vi "sequenceJsonIndex.vi"(8 "error in":errorcluster, 10 "StreamCluster":T1={"DAQ"={"ManagmentRate_Hz"=1, "StreamRate_Hz"=50, "StreamRate_ms"=20, "ManagmentRate_ms"=1000, "refDesArray"=[]}, "Modules"=[]}, 11 "JSON in":string) -> (0 "error out":errorcluster, 1 "refDes":string, 2 "cmd subset index":i32, 3 "cmd set index":i32)   [LabVIEW 2024]
uses:
  Control/StreamCluster_TypeDef.ctl
  c49e8bee-f697-436e-a8eb-f13d28c7991d.vi
  <vilib>/JDP Science/JSONtext/Find Item.vi
  <vilib>/JDP Science/JSONtext/Next JSON Value.vi
  <vilib>/JDP Science/JSONtext/String Subset.vi
  <vilib>/JDP Science/JSONtext/Parsing/Advance past next JSON Value (inlined COPY).vi
  <vilib>/JDP Science/JSONtext/Parsing/Advance past whitespace.vi
  <vilib>/JDP Science/JSONtext/Parsing/Advance past String.vi
  <vilib>/JDP Science/JSONtext/Parsing/Advance past Number.vi
  <vilib>/JDP Science/JSONtext/Parsing/Advance past Line Ending.vi
  <vilib>/JDP Science/JSONtext/Parsing/Parse Full Path or Item Name.vi
  <vilib>/JDP Science/JSONtext/Parsing/Advance past Array.vi
  <vilib>/JDP Science/JSONtext/Parsing/Advance past Object.vi
  <vilib>/JDP Science/JSONtext/support/Error Cluster From Code.vi
  <vilib>/JDP Science/JSONtext/Offset/Find Item Locations by Path.vi
  <vilib>/JDP Science/JSONtext/JSON text to Variant.vi
  <vilib>/JDP Science/JSONtext/LVClass Serializer/JSONtext LVClass Serializer.lvclass
  <vilib>/ErrorRing/Error Ring.xnode
  <vilib>/Utility/error.llb/Error Cluster From Error Code.vi
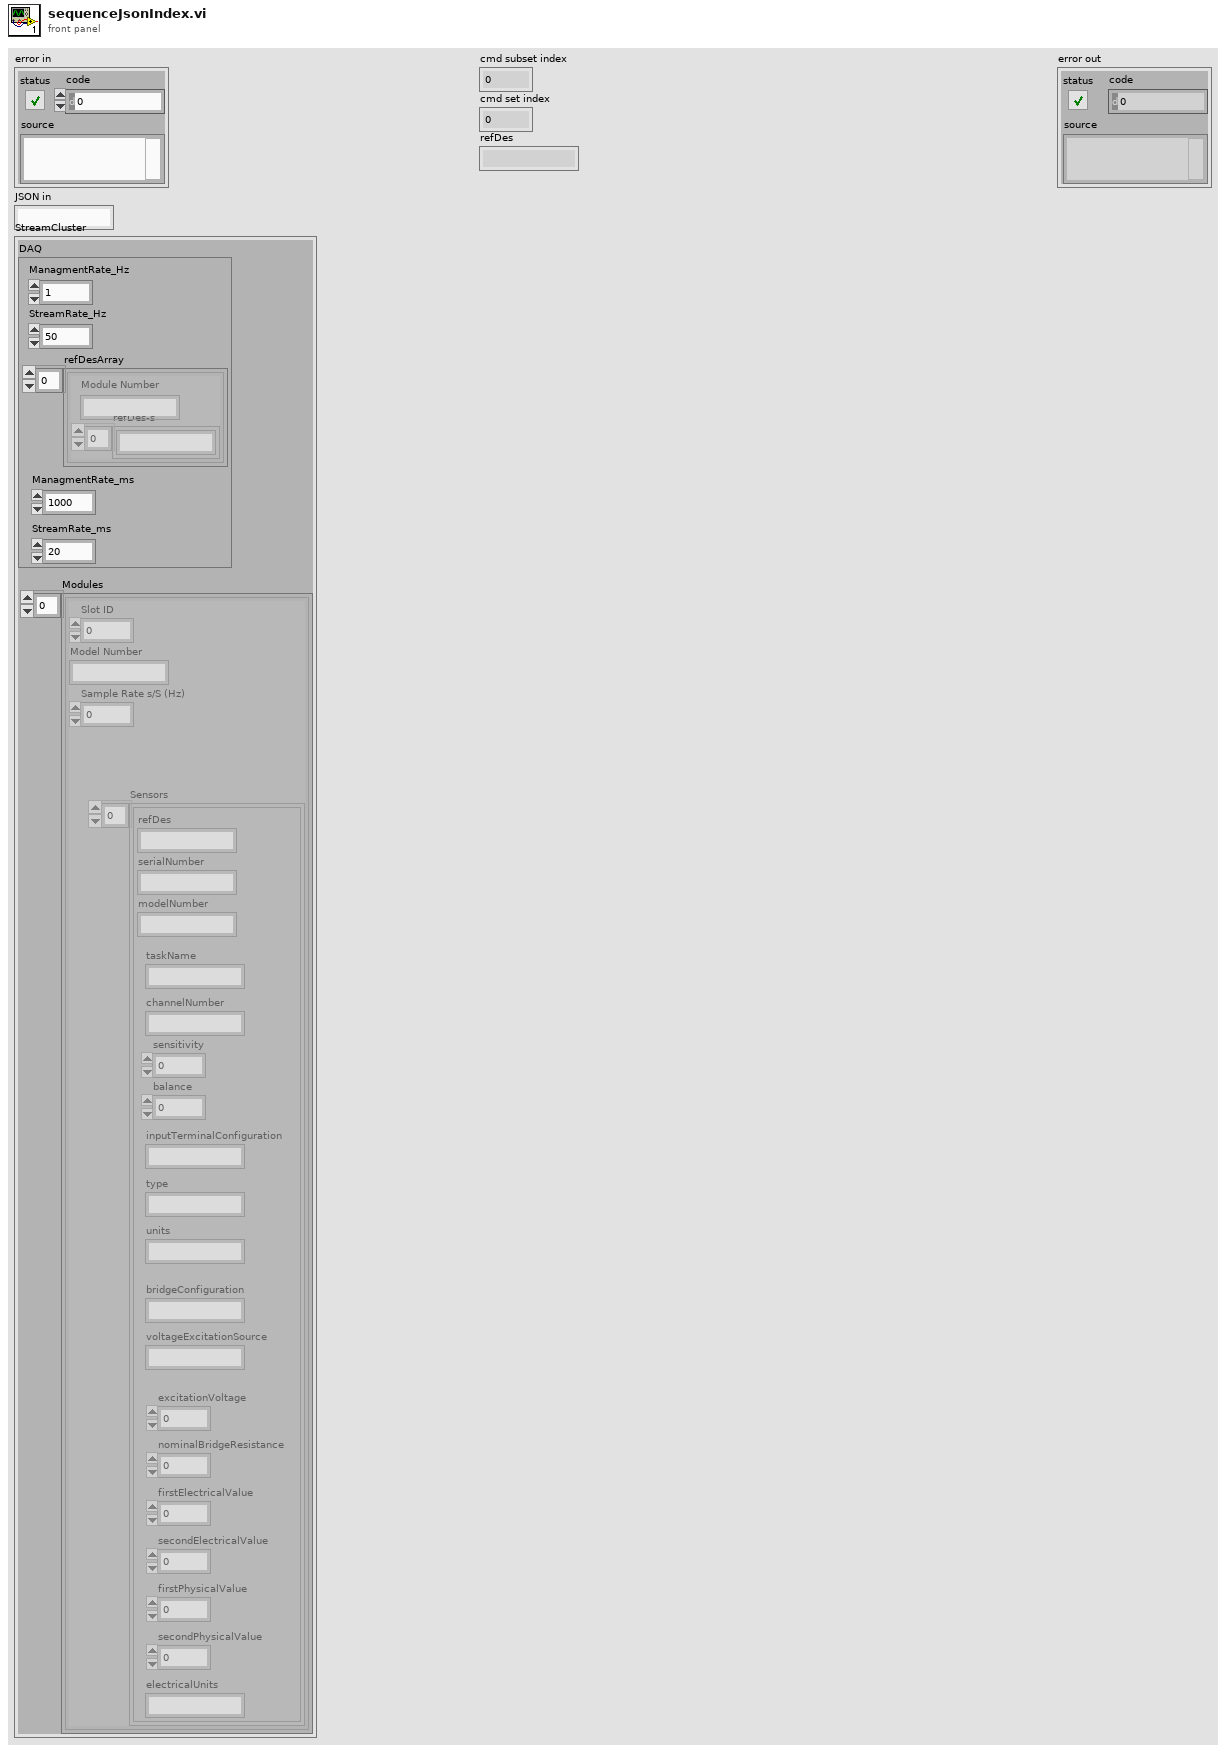
[diagram p1: front panel]
types:
  T1 = typedef "StreamCluster_TypeDef.ctl" = cluster{"DAQ":cluster{"ManagmentRate_Hz":i32, "StreamRate_Hz":i32, "StreamRate_ms":i32, "ManagmentRate_ms":i32, "refDesArray":cluster{"refDes-s":string[], "Module Number":string}[]}, "Modules":cluster{"Slot ID":i32, "Model Number":string, "Sample Rate s/S (Hz)":dbl, "Sensors":cluster{"refDes":string, "serialNumber":string, "modelNumber":string, "units":string, "balance":dbl, "sensitivity":dbl, "type":string, "inputTerminalConfiguration":string, "channelNumber":string, "taskName":string, "bridgeConfiguration":string, "excitationVoltage":dbl, "voltageExcitationSource":string, "nominalBridgeResistance":dbl, "firstElectricalValue":dbl, "secondElectricalValue":dbl, "firstPhysicalValue":dbl, "secondPhysicalValue":dbl, "electricalUnits":string}[]}[]}
  T2 = cluster{"refDes-s":string[], "Module Number":string}[]
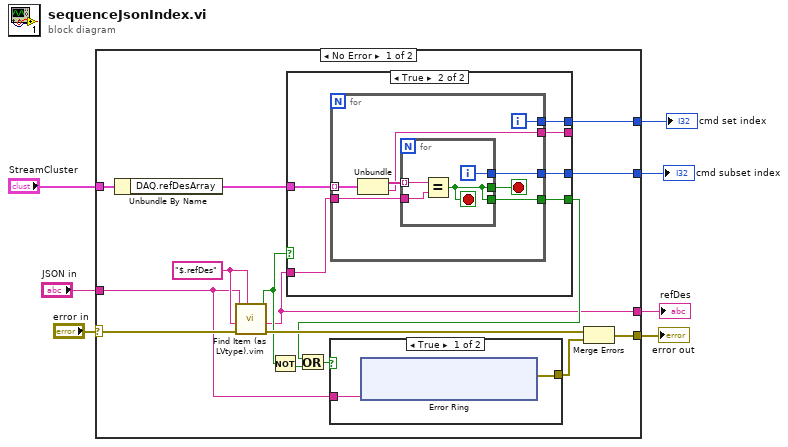
[diagram p0: block diagram]
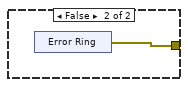
[diagram p2: hidden frame]
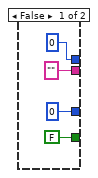
[diagram p3: hidden frame]
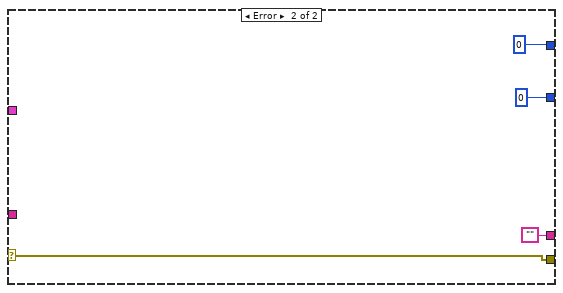
[diagram p4: hidden frame]
diagram:
  n1 = case shown="No Error" "error in" {
    selector: "error in" -> [w21 w59]
    tunnel: [w18 w59] -> w6
    tunnel: "JSON in" -> [w13 _]
    tunnel: "StreamCluster" -> [w20 _]
    tunnel: [w16 0] -> w3
    tunnel: [w15 0] -> w2
    tunnel: [w8 ""] -> w1
    frame No Error {
      w22 = "$.refDes" ("$Path or Item Name")
      n2 = Unbundle By Name(w20) -> ("DAQ.refDesArray"=w17:T2)
      n3 = call "Find Item (as LVtype).vim"("$Path or Item Name"=w22, "error in (no error)"=w21, "Data Type and Default Value"=w22, "JSON"=w13) -> ("error out"=w19:errorcluster, "Data"=w8:string, "Found"=w12:bool)  [unwired: 4 in, 1 out]
      n4 = Not(x=w12) -> (.not. x?=w10:bool)
      n5 = case shown="True" w12 {
        tunnel: w8 -> [_ w43]
        tunnel: w17 -> [_ w42]
        tunnel: [0 w41] -> w16
        tunnel: [0 w40] -> w15
        tunnel: [FALSE w39] -> w9
        tunnel: ["" ("Module Number") w38] -> _
        frame False {
        }
        frame True {
          n6 = for {
            tunnel: w43 -> [w49]
            tunnel: w42 -> [w51] mode=indexing
            tunnel: [w47] -> w39
            tunnel: [w46] -> w41
            tunnel: [w45] -> w40
            tunnel: [w44] -> w38
            i -> [w45]
            stop <- w48 stop-if-true
            n7 = Unbundle(w51) -> ("refDes-s"=w50:string[], "Module Number"=w44:string)
            n8 = for {
              tunnel: w50 -> [w55] mode=indexing
              tunnel: w49 -> [w54]
              tunnel: [w53] -> w48
              tunnel: [w53] -> w47
              tunnel: [w52] -> w46
              i -> [w52]
              stop <- w53 stop-if-true
              n9 = Equal?(x=w55, y=w54) -> (x = y?=w53:bool)
            }
          }
        }
      }
      n10 = Or(x=w9, y=w10) -> (x .or. y?=w11:bool)
      n11 = case shown="True" w11 {
        tunnel: [w24 w32] -> w14
        tunnel: w13 -> [w23 _]
        frame True {
          n12 = xnode "Error Ring"("parameter 0"=w23) -> ("error out"=w24:errorcluster)
        }
        frame False {
          n13 = xnode "Error Ring"() -> ("error out"=w32:errorcluster)
        }
      }
      n14 = Merge Errors(w19, w14) -> (w18:errorcluster)
    }
    frame Error {
    }
  }
  "error out" <- w6
  "cmd subset index" <- w3
  "cmd set index" <- w2
  "refDes" <- w1
